vi "solar_excel Workbook Close.vi"(8 "error in (no error)":errorcluster, 9 "Save? (F)":bool, 10 "Excel Workbook (*.xlsx)":path, 11 "Excel Workbook":T2) -> (0 "error out":errorcluster, 3 "Excel App":T1)   [LabVIEW 2018]
doc: "This closes a Workbook reference and returns the Excel Application reference. <b>Excel Workbook</b> must be specified if <b>Save?</b> is true."
uses:
  solar_excel_ctl App.ctl
  solar_excel_ctl TSV.ctl
  solar_excel_ctl Workbook.ctl
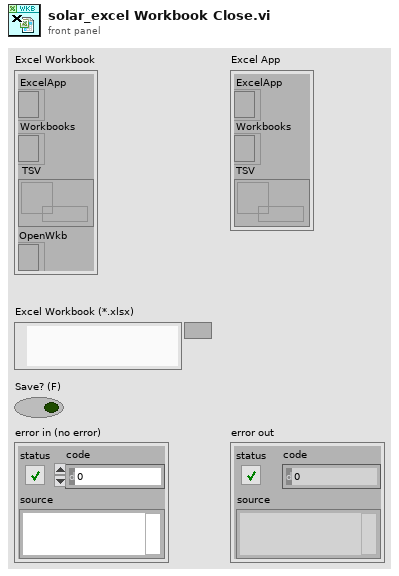
[diagram p1: front panel]
types:
  T1 = typedef "solar_excel_ctl App.ctl" = cluster{"ExcelApp":refnum<k7>, "Workbooks":refnum<k7>, "TSV":refnum<queue>}
  T2 = typedef "solar_excel_ctl Workbook.ctl" = cluster{"ExcelApp":refnum<k7>, "Workbooks":refnum<k7>, "TSV":refnum<queue>, "OpenWkb":refnum<k7>}
  T3 = typedef "solar_excel_ctl TSV.ctl" = cluster{"Path":path, "Dirty":bool, "ActiveSheet":u8, "Worksheets":string[], "Worksheet Cells":cluster{"Cells":string[][]}[]}
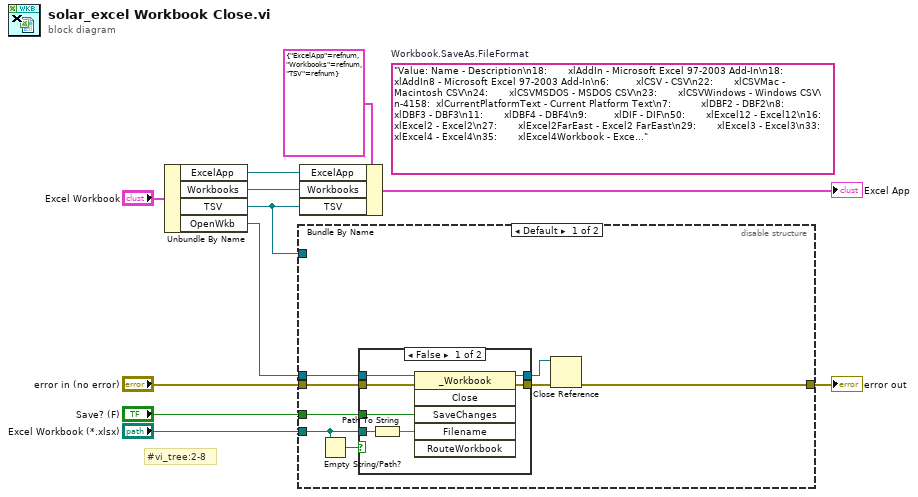
[diagram p0: block diagram]
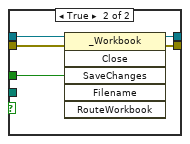
[diagram p2: hidden frame]
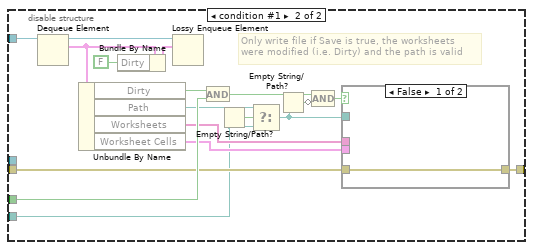
[diagram p3: hidden frame]
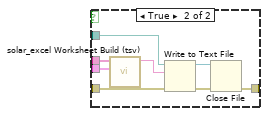
[diagram p4: hidden frame]
diagram:
  (unwired) "Value: Name - Description\n18:       xlAddIn - Microsoft Excel 97-2003 Add-In\n18:       xlAddIn8 - Microsoft Excel 97-2003 Add-In\n6:         xlCSV - CSV\n22:       xlCSVMac - Macintosh CSV\n24:       xlCSVMSDOS - MSDOS CSV\n23:       xlCSVWindows - Windows CSV\n-4158:  xlCurrentPlatformText - Current Platform Text\n7:          xlDBF2 - DBF2\n8:          xlDBF3 - DBF3\n11:       xlDBF4 - DBF4\n9:         xlDIF - DIF\n50:       xlExcel12 - Excel12\n16:       xlExcel2 - Excel2\n27:       xlExcel2FarEast - Excel2 FarEast\n29:       xlExcel3 - Excel3\n33:       xlExcel4 - Excel4\n35:       xlExcel4Workbook - Excel4 Workbook\n39:       xlExcel5 - Excel5\n39:       xlExcel7 - Excel7\n56:       xlExcel8 - Excel8\n43:       xlExcel9795 - Excel9795\n44:       xlHtml - HTML format\n26:       xlIntlAddIn - International Add-In\n25:       xlIntlMacro - International Macro\n60:       xlOpenDocumentSpreadsheet - OpenDocument Spreadsheet\n55:       xlOpenXMLAddIn - Open XML Add-In\n61:       xlOpenXMLStrictWorkbook - Strict Open XML file\n54:       xlOpenXMLTemplate - Open XML Template\n53:       xlOpenXMLTemplateMacroEnabled - Open XML Template Macro Enabled\n51:       xlOpenXMLWorkbook - Open XML Workbook\n52:       xlOpenXMLWorkbookMacroEnabled - Open XML Workbook Macro Enabled\n2:         xlSYLK - SYLK\n17:       xlTemplate - Template\n17:       xlTemplate8 - Template 8\n19:       xlTextMac - Macintosh Text\n21:       xlTextMSDOS - MSDOS Text\n36:       xlTextPrinter - Printer Text\n20:       xlTextWindows - Windows Text\n42:       xlUnicodeText - Unicode Text\n45:       xlWebArchive - Web Archive\n14:       xlWJ2WD1 - WJ2WD1\n40:       xlWJ3 - WJ3\n41:       xlWJ3FJ3 - WJ3FJ3\n5:         xlWK1 - WK1\n31:       xlWK1ALL - WK1ALL\n30:       xlWK1FMT - WK1FMT\n15:       xlWK3 - WK3\n32:       xlWK3FM3 - WK3FM3\n38:       xlWK4 - WK4\n4:         xlWKS - Worksheet\n51:       xlWorkbookDefault - Workbook default\n-4143: xlWorkbookNormal - Workbook normal\n28:       xlWorks2FarEast - Works2 FarEast\n34:       xlWQ1 - WQ1\n46:       xlXMLSpreadsheet - XML Spreadsheet"  # Workbook.SaveAs.FileFormat
  # "#vi_tree:2-8"
  n1 = Unbundle By Name("Excel Workbook") -> ("ExcelApp"=w10:refnum<k7>, "Workbooks"=w9:refnum<k7>, "TSV"=w1:refnum<queue>, "OpenWkb"=w7:refnum<k7>)
  n2 = disable-structure shown="Default" {
    disable-tunnel: "error in (no error)" -> [w18 w42]
    disable-tunnel: w7 -> [w17 _]
    disable-tunnel: "Save? (F)" -> [w16 w46]
    disable-tunnel: [w15 w41] -> w5
    disable-tunnel: "Excel Workbook (*.xlsx)" -> [w13 w36]
    disable-tunnel: w1 -> [_ w49]
    frame condition #0 (active) {
      n3 = Empty String/Path?(string/path=w13) -> (empty?=w12:bool)
      n4 = case shown="False" w12 {
        tunnel: [w26 w31] -> w19
        tunnel: w18 -> [w25 w30]
        tunnel: w17 -> [w24 w29]
        tunnel: w16 -> [w23 w28]
        tunnel: [w22 w27] -> w14
        tunnel: w13 -> [w21 _]
        frame False {
          n5 = Path To String(path=w21) -> (string=w20:string)
          n6 = invoke class="_Workbook" method="Close"(reference=w24, error in=w25, "SaveChanges"=w23, "Filename"=w20) -> (reference out=w22:refnum<k7>, error out=w26:errorcluster)  [unwired: 2 in, 4 out]
        }
        frame True {
          n7 = invoke class="_Workbook" method="Close"(reference=w29, error in=w30, "SaveChanges"=w28) -> (reference out=w27:refnum<k7>, error out=w31:errorcluster)  [unwired: 3 in, 4 out]
        }
      }
      n8 = Close Reference(reference=w14, error in (no error)=w19) -> (error out=w15:errorcluster)
    }
    frame condition #1 {
      # "Only write file if Save is true, the worksheets\nwere modified (i.e. Dirty) and the path is valid"
      n9 = Dequeue Element(queue=w49) -> (queue out=w48:refnum<queue>, element=w47:T3)  [unwired: 2 in, 2 out]
      n10 = Unbundle By Name(w47) -> ("Dirty"=w45:bool, "Path"=w37:path, "Worksheets"=w40:string[], "Worksheet Cells"=w39:cluster{"Cells":string[][]}[])
      n11 = Bundle By Name(cluster=w47, "Dirty"=FALSE) -> (w44:T3)
      n12 = Lossy Enqueue Element(queue=w48, element=w44) -> ()  [unwired: 1 in, 4 out]
      n13 = And(x=w45, y=w46) -> (x .and. y?=w34:bool)
      n14 = Empty String/Path?(string/path=w36) -> (empty?=w38:bool)
      n15 = Select(t=w37, s=w38, f=w36) -> (s? t:f=w32:path)
      n16 = Empty String/Path?(string/path=w32) -> (empty?=w35:bool)
      n17 = Compound Arithmetic op=AND(w34, invert w35) -> (w33:bool)
      n18 = case shown="False" w33 {
        tunnel: w42 -> [w50 w57]
        tunnel: [w50 w56] -> w41
        tunnel: w40 -> [_ w55]
        tunnel: w39 -> [_ w54]
        tunnel: w32 -> [_ w51]
        frame False {
        }
        frame True {
          n19 = call "solar_excel Worksheet Build (tsv).vi"("Worksheets Cells"=w54, "Worksheets"=w55) -> ("Tab Delimited String"=w58:string)  [unwired: 9 in]
          n20 = Write to Text File(file (use dialog)=w51, text=w58, error in=w57) -> (refnum out=w52:refnum<file>, error out=w53:errorcluster)  [unwired: 1 in, 1 out]
          n21 = Close File(refnum=w52, error in=w53) -> (error out=w56:errorcluster)  [unwired: 1 out]
        }
      }
    }
  }
  "error out" <- w5
  n22 = Bundle By Name(cluster=T1 {"ExcelApp"=refnum, "Workbooks"=refnum, "TSV"=refnum} ("Excel App 2"), "ExcelApp"=w10, "Workbooks"=w9, "TSV"=w1) -> (→"Excel App":T1)
